vi "Find Grey.vi"(8 "error in (no error)":errorcluster, 10 "Grey Index (0-255)":u8, 11 "ColorSelector in":refnum<class "ColorSelector.lvclass">) -> (0 "error out":errorcluster, 3 "ColorSelector out":refnum<class "ColorSelector.lvclass">)   [LabVIEW 2015, in "ColorSelector.lvclass"]
doc: "This VI finds the closest grey in the Grey Selector.\n<b> </b> <b> </b>\n©2017 Q Software Innovations, LLC (QSI)\nwritten by Quentin Alldredge\nproduced in LabVIEW 2015\n\nsupport@qsoftwareinnovations.com\nwww.qsoftwareinnovations.com\n\nAll rights reserved.\n\nRedistribution and use in source and binary forms, with or without modification, are permitted provided that the following conditions are met:\n\n * Redistributions of source code must retain the above copyright notice, this list of conditions and the following disclaimer.\n * Redistributions in binary form must reproduce the above copyright notice, this list of conditions and the following disclaimer in the documentation and/or other materials provided with the distribution.\n * Neither the name of Q Software Innovations, LLC. nor the names of its contributors may be used to endorse or promote products derived from this software without specific prior written permission.\n\nTHIS SOFTWARE IS PROVIDED BY THE COPYRIGHT HOLDERS AND CONTRIBUTORS \"AS IS\" AND ANY EXPRESS OR IMPLIED WARRANTIES, INCLUDING, BUT NOT LIMITED TO, THE IMPLIED WARRANTIES OF MERCHANTABILITY AND FITNESS FOR A PARTICULAR PURPOSE ARE DISCLAIMED. IN NO EVENT SHALL THE COPYRIGHT OWNER OR CONTRIBUTORS BE LIABLE FOR ANY DIRECT, INDIRECT, INCIDENTAL, SPECIAL, EXEMPLARY, OR CONSEQUENTIAL DAMAGES (INCLUDING, BUT NOT LIMITED TO, PROCUREMENT OF SUBSTITUTE GOODS OR SERVICES; LOSS OF USE, DATA, OR PROFITS; OR BUSINESS INTERRUPTION) HOWEVER CAUSED AND ON ANY THEORY OF LIABILITY, WHETHER IN CONTRACT, STRICT LIABILITY, OR TORT (INCLUDING NEGLIGENCE OR OTHERWISE) ARISING IN ANY WAY OUT OF THE USE OF THIS SOFTWARE, EVEN IF ADVISED OF THE POSSIBILITY OF SUCH DAMAGE."
uses:
  ColorSelector.lvclass
  <vilib>/Utility/miscctls.llb/LVPoint32TypeDef.ctl
  Read GreySelectPic.vi
  Write GreyGridCoords.vi
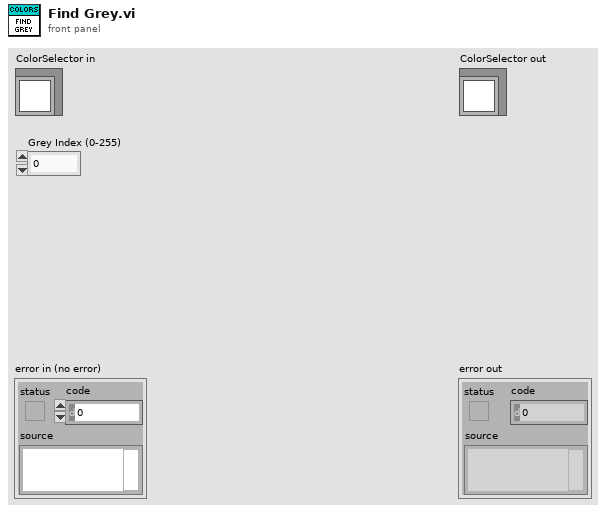
[diagram p1: front panel]
types:
  T1 = typedef "LVPoint32TypeDef.ctl" = cluster{"Horizontal":i32, "Vertical":i32}
  T2 = typedef "imagedata.ctl" = cluster{"image type":i32, "image depth":i32, "image":u8[], "mask":u8[], "colors":u32[], "Rectangle":cluster{"left":i16, "top":i16, "right":i16, "bottom":i16}}
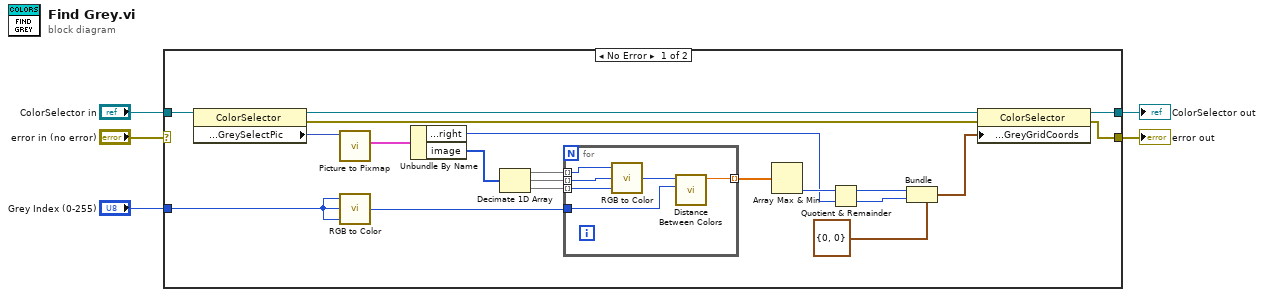
[diagram p0: block diagram]
diagram:
  n1 = case shown="No Error" "error in (no error)" {
    selector: "error in (no error)" -> [_ w33]
    tunnel: [w8 w33] -> w4
    tunnel: [w14 w32] -> w2
    tunnel: "ColorSelector in" -> [w25 w32]
    tunnel: "Grey Index (0-255)" -> [w7 _]
    frame No Error {
      n2 = property class="ColorSelector"(reference=w25) -> (reference out=w24:refnum<class "ColorSelector.lvclass">, error out=w9:errorcluster, "State Data:Accessors:GreySelectPic"=w23:picture)  [unwired: 1 in]
      n3 = call <vilib>:"Picture to Pixmap.vi"("picture"=w23) -> ("image data"=w22:T2)  [unwired: 9 in, 1 out]
      n4 = call <vilib>:"RGB to Color.vi"("B"=w7, "G"=w7, "R"=w7) -> ("Color"=w6:u32)
      n5 = Unbundle By Name(w22) -> ("Rectangle.right"=w15:i16, "image"=w16:u8[])
      n6 = Decimate 1D Array(w16) -> (w17:u8[], w18:u8[], w19:u8[])
      n7 = for {
        tunnel: w17 -> [w29] mode=indexing
        tunnel: w18 -> [w30] mode=indexing
        tunnel: w19 -> [w31] mode=indexing
        tunnel: w6 -> [w27]
        tunnel: [w26] -> w20 mode=indexing
        n8 = call <vilib>:"RGB to Color.vi"("B"=w31, "G"=w30, "R"=w29) -> ("Color"=w28:u32)
        n9 = call "Distance Between Colors.vi"("Color 2"=w27, "Color 1"=w28) -> ("Distance"=w26:dbl)  [unwired: 8 in, 1 out]
      }
      n10 = Array Max & Min(array=w20) -> (min index (indices)=w21:i32)  [unwired: 3 out]
      n11 = Quotient & Remainder(x=w21, y=w15) -> (x-y*floor(x/y)=w12:i32, floor(x/y)=w11:i32)
      n12 = Bundle(cluster=T1 {"Horizontal"=0, "Vertical"=0} ("ColorGridCoords"), "Horizontal"=w12, "Vertical"=w11) -> (w10:T1)
      n13 = property class="ColorSelector"(reference=w24, error in=w9, "State Data:Accessors:GreyGridCoords"=w10) -> (reference out=w14:refnum<class "ColorSelector.lvclass">, error out=w8:errorcluster)
    }
    frame Error {
    }
  }
  "error out" <- w4
  "ColorSelector out" <- w2
